vi "Elapsed Time.vi"(8 "error in":errorcluster, 9 "timeout (ms)":u32, 11 "past time":u32) -> (0 "error out":errorcluster, 1 "Timeout?":bool, 2 "elapsed time (ms)":u32, 3 "millisecond timer value":u32, 4 "Elapsed Time String":string)   [LabVIEW 2023]
doc: "Reuse this on a Block diagram to time points in code execution. The elapsed time is the difference between current time and last time."
uses:
  <userlib>/_OpenG.lib/time/time.llb/openg_time.lvlib
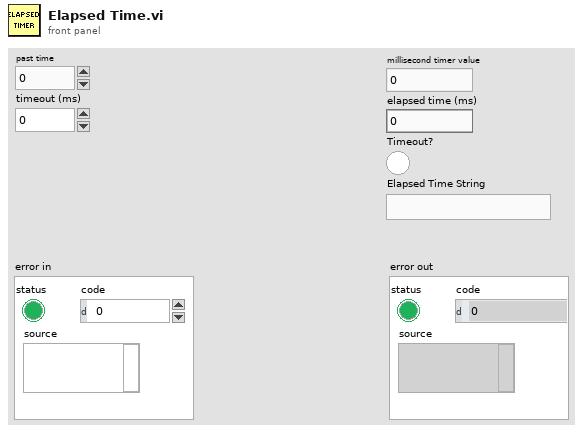
[diagram p1: front panel]
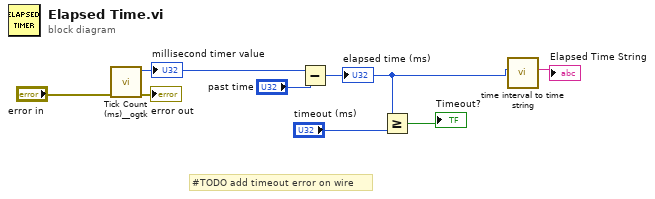
[diagram p0: block diagram]
diagram:
  # "#TODO add timeout error on wire"
  n1 = call <userlib>:"Tick Count (ms)__ogtk.vi"("error in (no error)"="error in") -> ("error out"=→"error out":errorcluster, "millisecond timer value"=w6:u32)  [unwired: 9 in]
  "millisecond timer value" <- w6
  n2 = Subtract(x=w6, y="past time") -> (x-y=w2:u32)
  "elapsed time (ms)" <- w2
  n3 = Greater Or Equal?(x=w2, y="timeout (ms)") -> (x >= y?=→"Timeout?":bool)
  n4 = call "time interval to time string.vi"("time interval"=w2) -> ("Time String"=→"Elapsed Time String":string)  [unwired: 4 in]
